vi "Get_INI_Calibrator_Section.vi"(0 "Sequence Path":path, 1 "name or relative path":string="ModisEdge.ini", 2 "section":string="Calibrator", 3 "error in (no error)":errorcluster) -> (6 "Delay(s)":i32, 9 "error out":errorcluster)   [LabVIEW 2015]
uses:
  <vilib>/Utility/config.llb/Read Key (I32).vi
  <vilib>/Utility/config.llb/NI_LVConfig.lvlib
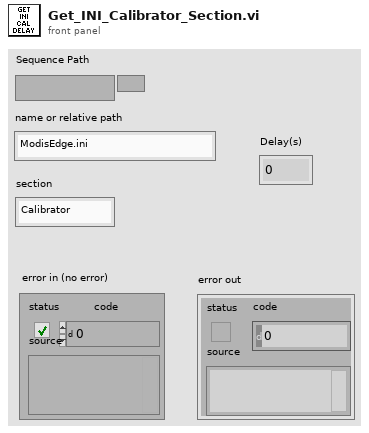
[diagram p1: front panel]
types:
  T1 = typedef "NI_LVConfig.lvlib/Config Data RefNum.ctl" = refnum<k1>
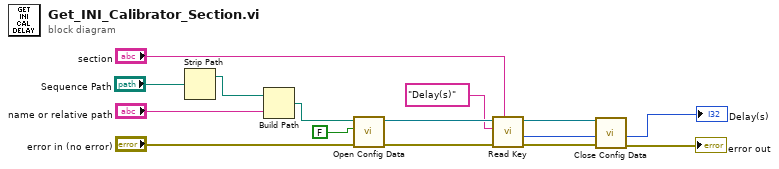
[diagram p0: block diagram]
diagram:
  n1 = Strip Path(path="Sequence Path") -> (stripped path=w1:path)  [unwired: 1 out]
  n2 = Build Path(base path=w1, name or relative path="name or relative path") -> (appended path=w7:path)
  n3 = call <vilib>:"Open Config Data.vi"("error in (no error)"="error in (no error)", "create file if necessary (T)"=FALSE, "configuration file path"=w7) -> ("error out"=w6:errorcluster, "refnum"=w5:T1)  [unwired: 6 in, 1 out]
  n4 = call-poly <vilib>:"Read Key.vi"("section"="section", "error in (no error)"=w6, "key"="Delay(s)", "refnum"=w5) -> ("error out"=w12:errorcluster, "value"=→"Delay(s)":i32, "refnum out"=w11:T1)  [unwired: 4 in, 1 out]
  n5 = call <vilib>:"Close Config Data.vi"("error in (no error)"=w12, "refnum"=w11) -> ("error out"=→"error out":errorcluster)  [unwired: 8 in, 1 out]
